vi "Run_Gnuplot_Script.vi"(0 "OutputType":enum16{"PDF", "PNG-ReportStyle"}(ring), 1 "logfileName":string, 2 "workingDirectory":path) -> ()   [LabVIEW 2014]
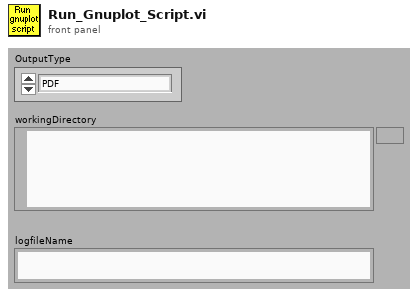
[diagram p1: front panel]
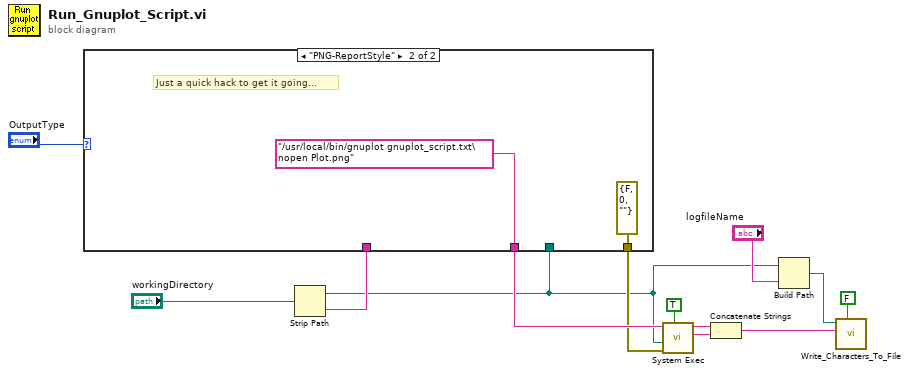
[diagram p0: block diagram]
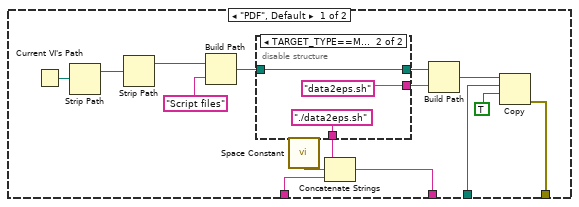
[diagram p2: hidden frame]
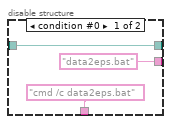
[diagram p3: hidden frame]
diagram:
  n1 = Strip Path(path="workingDirectory") -> (stripped path=w3:path, name=w7:string)
  n2 = case shown="\"PNG-ReportStyle\"" "OutputType" {
    tunnel: [w21 "/usr/local/bin/gnuplot gnuplot_script.txt\nopen Plot.png"] -> w8
    tunnel: w7 -> [w16 _]
    tunnel: [w15 errorcluster {"status"=FALSE, "code"=0, "source"=""} ("error out")] -> w6
    tunnel: w3 -> [w14 _]
    frame "PDF", Default {
      n3 = Current VI's Path() -> (path=w28:path)
      n4 = Strip Path(path=w28) -> (stripped path=w27:path)  [unwired: 1 out]
      n5 = Strip Path(path=w27) -> (stripped path=w26:path)  [unwired: 1 out]
      n6 = Build Path(base path=w26, name or relative path="Script files") -> (appended path=w24:path)
      n7 = disable-structure shown="TARGET_TYPE==Mac, Default" {
        disable-tunnel: w24 -> [w29 w34]
        disable-tunnel: [w29 w34] -> w20
        disable-tunnel: ["data2eps.bat" "data2eps.sh"] -> w19
        disable-tunnel: ["cmd /c data2eps.bat" "./data2eps.sh"] -> w17
        frame condition #0 {
        }
        frame condition #1 (active) {
        }
      }
      n8 = call <vilib>:"Space Constant.vi"() -> ("String"=w22:string)
      n9 = Concatenate Strings(w17, w22, w16) -> (w21:string)
      n10 = Build Path(base path=w20, name or relative path=w19) -> (appended path=w18:path)
      n11 = Copy(9:TRUE ("overwrite (F)"), 10:w14, 11:w18) -> (0:w15:errorcluster)  [unwired: 1 in, 3 out]
    }
    frame "PNG-ReportStyle" {
      # "Just a quick hack to get it going..."
    }
  }
  n12 = call <vilib>:"System Exec.vi"("wait until completion? (T)"=TRUE, "error in (no error)"=w6, "working directory"=w3, "command line"=w8) -> ("standard error"=w4:string, "standard output"=w12:string)  [unwired: 2 in, 4 out]
  n13 = Concatenate Strings(w12, w4) -> (w5:string)
  n14 = Build Path(base path=w3, name or relative path="logfileName") -> (appended path=w11:path)
  n15 = call "Write_Characters_To_File.vi"("file path (dialog if empty)"=w11, "advisory dialog? (display:T)"=FALSE, "character string"=w5) -> ()  [unwired: 2 in, 4 out]
